vi "GetTriggerSettings.vi"(8 "error in (no error)":errorcluster, 11 "T560Session in":refnum<class "T560Session.lvclass">) -> (0 "error out":errorcluster, 2 "TriggerSettings":T3, 3 "T560Session out":refnum<class "T560Session.lvclass">)   [LabVIEW 2020, in "T560Session.lvclass"]
doc: "Retrive the trigger settings from the Trigger object"
uses:
  T560Session.lvclass
  Common/TypeDefs/TriggerImpedance.ctl
  Common/TypeDefs/TriggerSource.ctl
  Common/TypeDefs/ChannelName.ctl
  T560TriggerClass/T560Trigger.lvclass
  C:/GEECS/Developers Version/source/Device Drivers/Highland T564 DDG/SupportLibraries/DeviceSpecific/HighlandT560Lib/T560ChannelClass/T560Channel.lvclass
  T560ChannelClass/T560Channel.lvclass
panel:
  out "Response":string
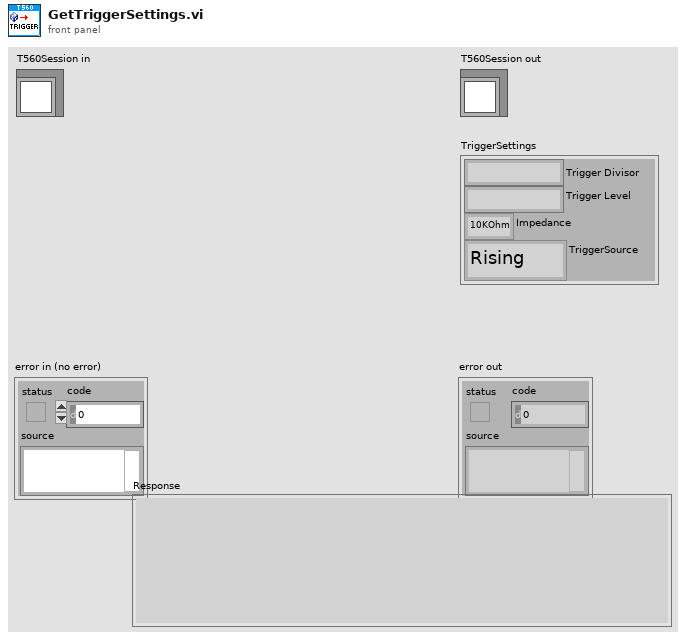
[diagram p1: front panel]
types:
  T1 = typedef "TriggerImpedance.ctl" = enum16{"10KOhm", "50Ohms"}
  T2 = typedef "TriggerSource.ctl" = enum16{"Rising", "Falling", "Internal 80MHz", "Internal DDS", "Remote", "Disabled"}
  T3 = cluster{"Trigger Divisor":string, "Trigger Level":string, "Impedance":T1, "TriggerSource":T2}
  T4 = typedef "T560Channel.lvclass/ChannelName.ctl" = enum16{"Null", "A", "B", "C", "D", "Trigger"}
  T5 = cluster{"PropertiesAccess:Trigger Divisor":string, "PropertiesAccess:Trigger Level":string, "PropertiesAccess:Impedance":enum16{"10KOhm", "50Ohms"}, "PropertiesAccess:TriggerSource":T2}
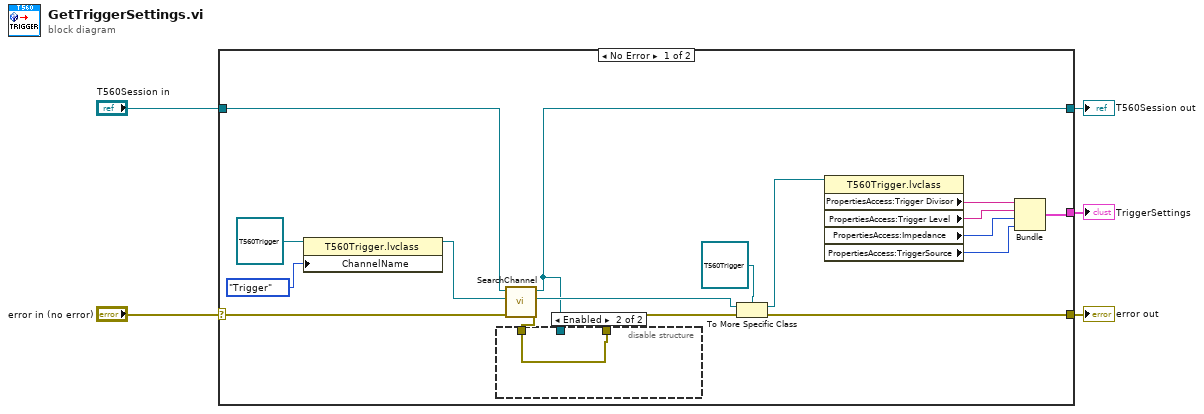
[diagram p0: block diagram]
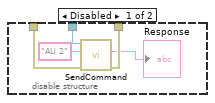
[diagram p2: hidden frame]
diagram:
  n1 = case shown="No Error" "error in (no error)" {
    selector: "error in (no error)" -> [w20 w30]
    tunnel: [w18 w30] -> w4
    tunnel: [w8 w29] -> w2
    tunnel: "T560Session in" -> [w22 w29]
    tunnel: [w10 _] -> w1
    frame No Error {
      n2 = property class="T560Trigger.lvclass"(reference=refnum<class "T560Trigger.lvclass"> refnum ("Highlandt564.lvlib:T560Trigger.lvclass"), "ChannelName"=ChannelName."Trigger") -> (reference out=w21:refnum<class "T560Trigger.lvclass">)  [unwired: 1 in, 1 out]
      n3 = call-dynamic "SearchChannel.vi"("error in"=w20, "T560Channel.lvclass"=w21, "T560Session in"=w22) -> ("error out"=w7:errorcluster, "T560Object.lvclass"=w9:refnum<class "T560Channel.lvclass">, "T560Session out"=w8:refnum<class "T560Session.lvclass">)  [unwired: 5 in, 1 out]
      n4 = disable-structure shown="Enabled" {
        disable-tunnel: w8 -> [w26 _]
        disable-tunnel: w7 -> [w25 w28]
        disable-tunnel: [w24 w28] -> w6
        frame Disabled {
          n5 = call-dynamic "SendCommand.vi"("error in"=w25, "Command"="AU 2", "T560Session in"=w26) -> ("error out"=w24:errorcluster, "Response"=→"Response":string)  [unwired: 6 in, 1 out]
        }
        frame Enabled {
        }
      }
      n6 = To More Specific Class(target class=refnum<class "T560Trigger.lvclass"> refnum ("Highlandt564.lvlib:T560Trigger.lvclass"), reference=w9, error in=w6) -> (specific class reference=w15:refnum<class "T560Trigger.lvclass">, error out=w18:errorcluster)
      n7 = property class="T560Trigger.lvclass"(reference=w15) -> ("PropertiesAccess:Trigger Divisor"=w14:string, "PropertiesAccess:Trigger Level"=w13:string, "PropertiesAccess:Impedance"=w12:enum16{"10KOhm", "50Ohms"}, "PropertiesAccess:TriggerSource"=w11:T2)  [unwired: 1 in, 2 out]
      n8 = Bundle("PropertiesAccess:Trigger Divisor"=w14, "PropertiesAccess:Trigger Level"=w13, "PropertiesAccess:Impedance"=w12, "PropertiesAccess:TriggerSource"=w11) -> (w10:T5)  [unwired: 1 in]
    }
    frame Error {
    }
  }
  "error out" <- w4
  "T560Session out" <- w2
  "TriggerSettings" <- w1
